vi "HexDisplayStringToHexString.vi"(11 "HEX显示字符串":string) -> (3 "正常显示HEX字符串":string)   [LabVIEW 2011]
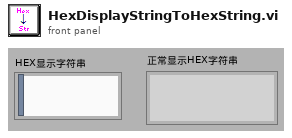
[diagram p1: front panel]
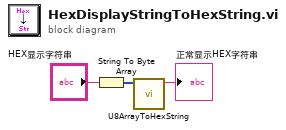
[diagram p0: block diagram]
diagram:
  n1 = String To Byte Array(string="HEX显示字符串") -> (unsigned byte array=w2:u8[])
  n2 = call "U8ArrayToHexString.vi"("u8 Data[]"=w2) -> ("HEX String (0-9,A-F)"=→"正常显示HEX字符串":string)  [unwired: 10 in]
